vi "TestsToJson.vi"(8 "error in (no error)":errorcluster, 11 "Test Array":refnum<class "TestInterface.lvclass">[](array[class])) -> (0 "error out":errorcluster, 3 "JSON string":string)   [LabVIEW 2013, in "DataCreation.lvlib"]
uses:
  classes/Tests/TestInterface/TestInterface.lvclass
  DataCreation.lvlib
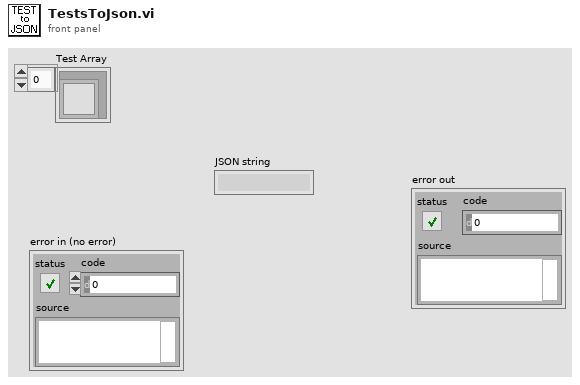
[diagram p1: front panel]
types:
  T1 = cluster{"class name":string, "Command regex":string[], "Commandlist":string, "name":string, "parameters":string[], "response":bool[], "timings":i32[], "wait":u32[]}
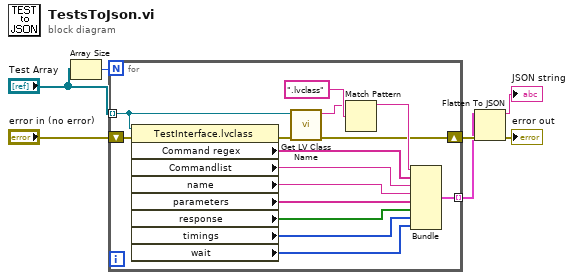
[diagram p0: block diagram]
diagram:
  n1 = Array Size(array="Test Array") -> (size(s)=w2:i32)
  n2 = for {
    N: w2 -> [_]
    tunnel: [w20] -> w5 mode=indexing
    tunnel: "Test Array" -> [w8] mode=indexing
    shift-right: [w21] -> w6
    shift-left: "error in (no error)" -> [w9]
    n3 = property class="TestInterface.lvclass"(reference=w8, error in=w9) -> (error out=w10:errorcluster, "Command regex"=w13:string[], "Commandlist"=w14:string, "name"=w15:string, "parameters"=w16:string[], "response"=w17:bool[], "timings"=w18:i32[], "wait"=w19:u32[])  [unwired: 1 out]
    n4 = call <vilib>:"Get LV Class Name.vi"("error in (no error)"=w10, "object"=w8) -> ("error out"=w21:errorcluster, "class name"=w11:string)  [unwired: 8 in]
    n5 = Match Pattern(string=w11, regular expression=".lvclass") -> (before substring=w22:string)  [unwired: 1 in, 3 out]
    n6 = Bundle("class name"=w22, "Command regex"=w13, "Commandlist"=w14, "name"=w15, "parameters"=w16, "response"=w17, "timings"=w18, "wait"=w19) -> (w20:T1)  [unwired: 1 in]
  }
  n7 = Flatten To JSON(anything=w5, error in (no error)=w6) -> (JSON string=→"JSON string":string, 11:→"error out":errorcluster)  [unwired: 1 in]
